vi "Spreadsheet String to Array.vi"(5 "Row Delimiter (;)":string=";", 7 "Sample Delimiter (,)":string=",", 11 "Spreadsheet String":string) -> (2 "1D Array":dbl[](array[numeric]), 3 "2D Array":dbl[][](array[numeric]))   [LabVIEW 2015, in "Neural Network.lvclass"]
uses:
  Neural Network.lvclass
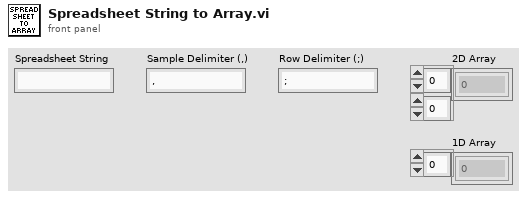
[diagram p1: front panel]
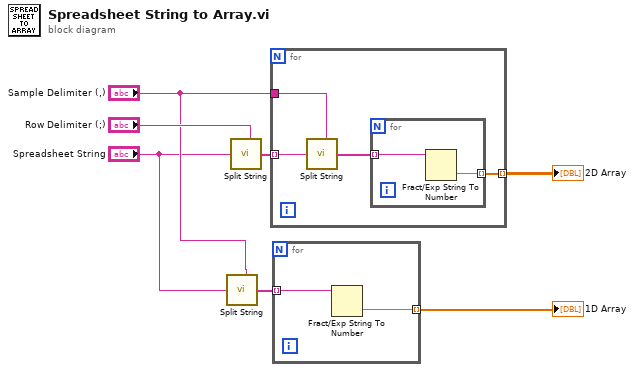
[diagram p0: block diagram]
diagram:
  n1 = call <vilib>:"Split String.vi"("Split Pattern"="Sample Delimiter (,)", "Input String"="Spreadsheet String") -> ("Split String"=w2:string[])  [unwired: 5 in]
  n2 = call <vilib>:"Split String.vi"("Split Pattern"="Row Delimiter (;)", "Input String"="Spreadsheet String") -> ("Split String"=w6:string[])  [unwired: 5 in]
  n3 = for {
    tunnel: w6 -> [w11] mode=indexing
    tunnel: [w9] -> w7 mode=indexing
    tunnel: "Sample Delimiter (,)" -> [w8]
    n4 = call <vilib>:"Split String.vi"("Split Pattern"=w8, "Input String"=w11) -> ("Split String"=w10:string[])  [unwired: 5 in]
    n5 = for {
      tunnel: w10 -> [w13] mode=indexing
      tunnel: [w12] -> w9 mode=indexing
      n6 = Fract/Exp String To Number(string=w13) -> (number=w12:dbl)  [unwired: 3 in, 1 out]
    }
  }
  "2D Array" <- w7
  n7 = for {
    tunnel: w2 -> [w15] mode=indexing
    tunnel: [w14] -> w1 mode=indexing
    n8 = Fract/Exp String To Number(string=w15) -> (number=w14:dbl)  [unwired: 3 in, 1 out]
  }
  "1D Array" <- w1
